vi "Read BIU Configuration.vi"(8 "error in":errorcluster, 11 "custom device":T1 format="%.0x") -> (0 "error out":errorcluster, 2 "biu configuration":T2, 3 "custom device out":T1 format="%.0x")   [LabVIEW 2020, in "AIM MIL-STD-1553 Scripting.lvlib"]
doc: "Returns bundled <b>biu configuration</b> information that was previously added to the specified <b>custom device</b>, including: \n1. Major Frames\n2. Minor Frames\n3. Acyclic Frame Names\n4. Terminal Names/Addresses\n5. Messages\n6. the Port Number (also called Hardware Channel)."
uses:
  AIM MIL-STD-1553 Scripting.lvlib
  <vilib>/NI VeriStand/Custom Device API/Custom Device Item Ref.ctl
  Shared/BIU Configuration.ctl
  Shared/Address.ctl
  Shared/Major Frame Definition.ctl
  Shared/Minor Frame Definition.ctl
  Shared/Acyclic Frame Definition.ctl
  Shared/Message Definition.ctl
  Shared/Message Type.ctl
  Shared/Terminal Endpoint.ctl
  Shared/Parameter Definition.ctl
  <vilib>/NI VeriStand/Custom Device API/Custom Device API.lvlib
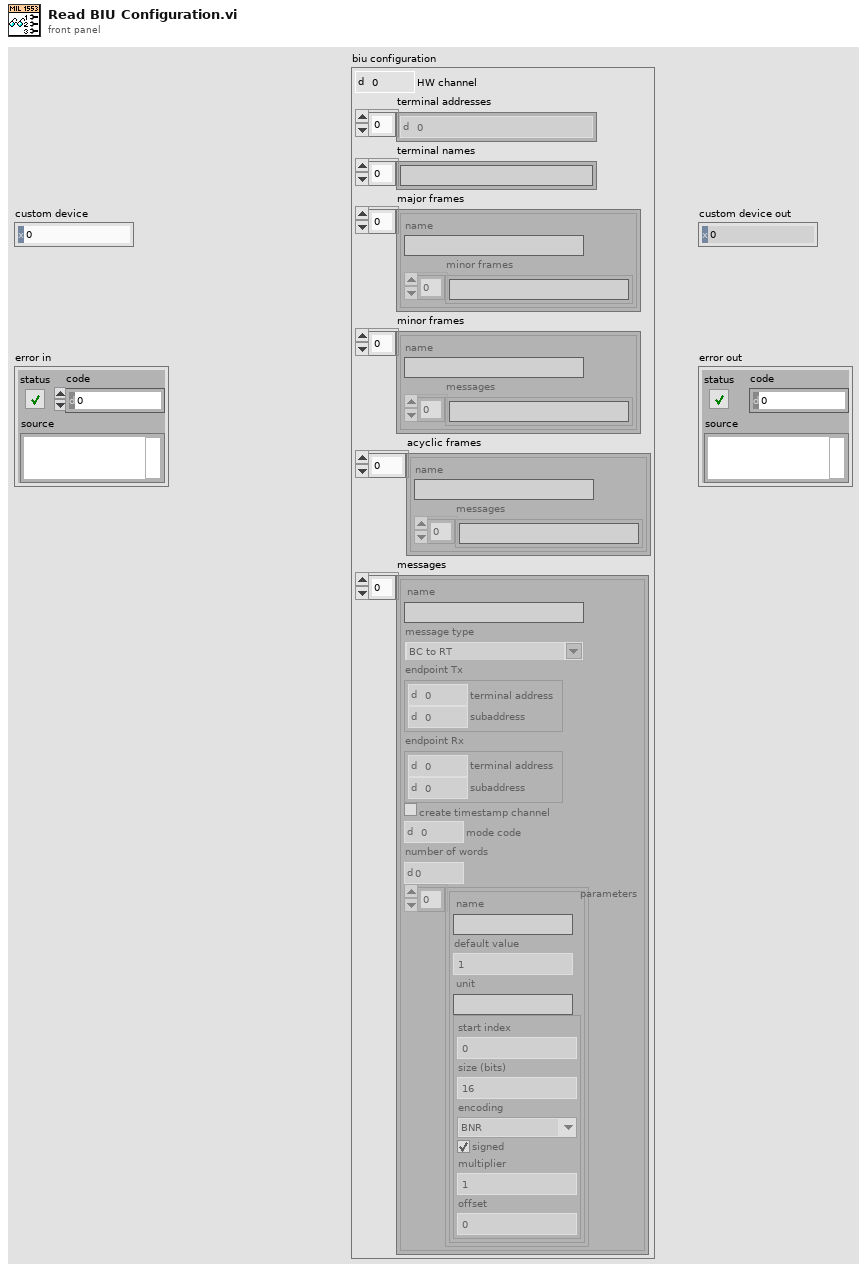
[diagram p1: front panel]
types:
  T1 = typedef "Custom Device API.lvlib/Custom Device Item Ref.ctl" = u64
  T2 = typedef "BIU Configuration.ctl" = cluster{"HW channel":u16, "terminal addresses":T3[], "terminal names":string[], "major frames":T4[], "minor frames":T5[], "acyclic frames":T6[], "messages":T7[]}
  T3 = typedef "Address.ctl" = u16
  T4 = typedef "Major Frame Definition.ctl" = cluster{"name":string, "minor frames":string[]}
  T5 = typedef "Minor Frame Definition.ctl" = cluster{"name":string, "messages":string[]}
  T6 = typedef "Acyclic Frame Definition.ctl" = cluster{"name":string, "messages":string[]}
  T7 = typedef "Message Definition.ctl" = cluster{"name":string, "message type":T8, "endpoint Tx":T9, "endpoint Rx":T9, "create timestamp channel":bool, "mode code":u16, "number of words":u16, "parameters":cluster{"name":string, "default value":dbl, "unit":string, "parameter definition":T10}[]}
  T8 = typedef "Message Type.ctl" = string
  T9 = typedef "Terminal Endpoint.ctl" = cluster{"terminal address":T3, "subaddress":T3}
  T10 = typedef "Parameter Definition.ctl" = cluster{"start index":i32, "size (bits)":i32, "encoding":enum16{"BNR", "BCD", "Discrete"}, "signed":bool, "multiplier":dbl, "offset":dbl}
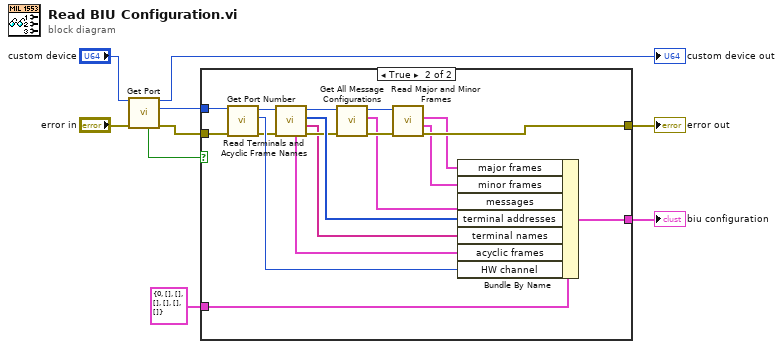
[diagram p0: block diagram]
diagram:
  n1 = call "Get Port.vi"("error in"="error in", "custom device ref"="custom device") -> ("error out"=w6:errorcluster, "port"=w5:T1, "custom device ref out"=→"custom device out":T1, "found"=w1:bool)  [unwired: 6 in]
  n2 = case shown="True" w1 {
    tunnel: [w11 w29] -> w9
    tunnel: w6 -> [w11 w28]
    tunnel: w5 -> [_ w27]
    tunnel: [w10 w26] -> w3
    tunnel: T2 {"HW channel"=0, "terminal addresses"=[], "terminal names"=[], "major frames"=[], "minor frames"=[], "acyclic frames"=[], "messages"=[]} ("1553 channel") -> [w10 w13]
    frame False {
      # "since no port, return the \ndefault configuration"
    }
    frame True {
      n3 = call "Get Port Number.vi"("error in"=w28, "port"=w27) -> ("error out"=w23:errorcluster, "port number"=w25:u16, "port out"=w24:T1)  [unwired: 6 in, 1 out]
      n4 = call "Read Terminals and Acyclic Frame Names.vi"("error in"=w23, "port"=w24) -> ("error out"=w20:errorcluster, "terminal names"=w17:string[], "terminals"=w22:T3[], "port out"=w21:T1, "acyclic frames"=w12:T6[])  [unwired: 5 in]
      n5 = call "Get All Message Configurations.vi"("error in"=w20, "port"=w21) -> ("error out"=w19:errorcluster, "message configurations"=w18:T7[], "port out"=w16:T1)  [unwired: 7 in]
      n6 = call "Read Major and Minor Frames.vi"("error in"=w19, "port"=w16) -> ("error out"=w29:errorcluster, "minor frames"=w14:T5[], "major frames"=w15:T4[])  [unwired: 6 in, 1 out]
      n7 = Bundle By Name(cluster=w13, "major frames"=w15, "minor frames"=w14, "messages"=w18, "terminal addresses"=w22, "terminal names"=w17, "acyclic frames"=w12, "HW channel"=w25) -> (w26:T2)
    }
  }
  "error out" <- w9
  "biu configuration" <- w3
